vi "Write Selection.vi"(8 "error in (no error)":errorcluster, 10 "Selection (-1: none)":i8=-1, 11 "Dialog_2Buttons.lvclass in":refnum<class "Dialog_TwoButtons.lvclass">) -> (0 "error out":errorcluster, 3 "Dialog_2Buttons.lvclass out":refnum<class "Dialog_TwoButtons.lvclass">)   [LabVIEW 2012, in "Dialog_TwoButtons.lvlib" / "Dialog_TwoButtons.lvclass"]
doc: "Accessor VI for Dialog_2Button class"
uses:
  Dialog_TwoButtons.lvclass
  Dialog_TwoButtons.lvclass/Dialog_TwoButtons.ctl
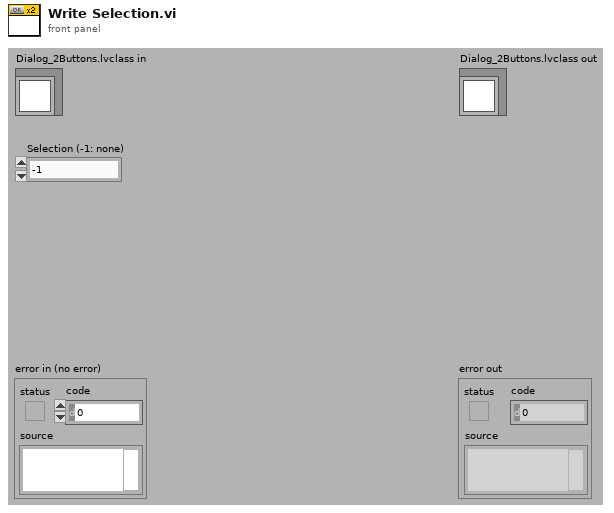
[diagram p1: front panel]
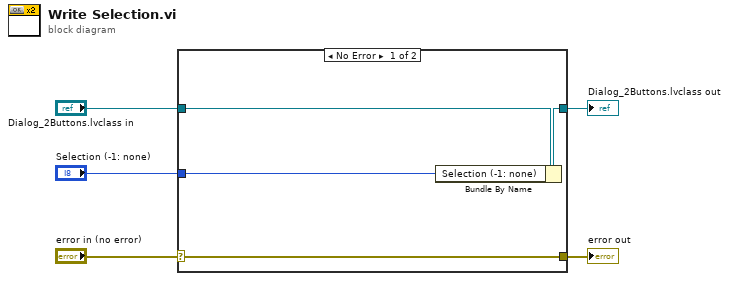
[diagram p0: block diagram]
diagram:
  n1 = case shown="No Error" "error in (no error)" {
    selector: "error in (no error)" -> [w9 w10]
    tunnel: [w9 w10] -> w4
    tunnel: [w7 w11] -> w2
    tunnel: "Dialog_2Buttons.lvclass in" -> [w8 w11]
    tunnel: "Selection (-1: none)" -> [w6 _]
    frame No Error {
      n2 = Bundle By Name(cluster=w8, "Selection (-1: none)"=w6) -> (w7:refnum<class "Dialog_TwoButtons.lvclass">)
    }
    frame Error {
    }
  }
  "error out" <- w4
  "Dialog_2Buttons.lvclass out" <- w2
